vi "reportResult_getEvent.vi"(8 "error in (no error)":errorcluster, 9 "timesSuccess":i32, 10 "timesTest":i32, 11 "SalProcess in":refnum<class "SalProcess.lvclass">) -> (0 "error out":errorcluster, 3 "SalProcess out":refnum<class "SalProcess.lvclass">)   [LabVIEW 2018, in "SalProcess.lvclass"]
doc: "Report the test result of getting the event."
uses:
  SalProcess.lvclass
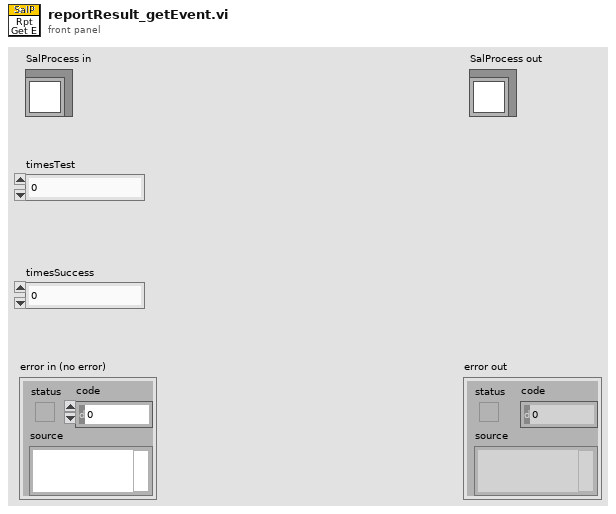
[diagram p1: front panel]
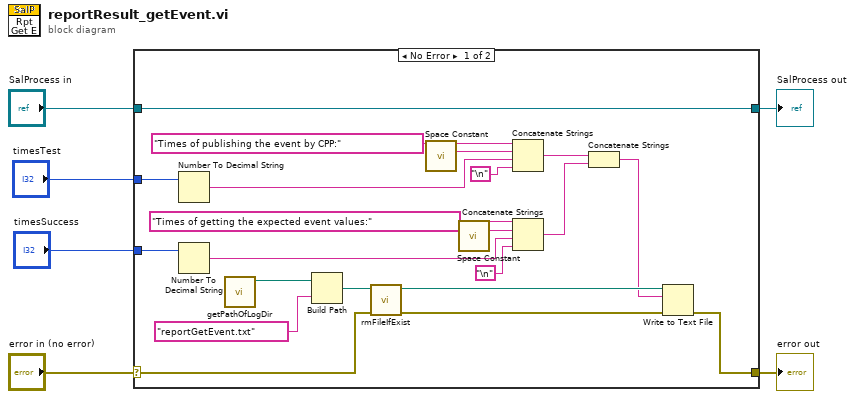
[diagram p0: block diagram]
diagram:
  n1 = case shown="No Error" "error in (no error)" {
    selector: "error in (no error)" -> [w23 w29]
    tunnel: [w7 w29] -> w5
    tunnel: [w27 w28] -> w3
    tunnel: "SalProcess in" -> [w27 w28]
    tunnel: "timesTest" -> [w22 _]
    tunnel: "timesSuccess" -> [w21 _]
    frame No Error {
      n2 = Number To Decimal String(number=w22) -> (decimal integer string=w18:string)  [unwired: 1 in]
      n3 = Number To Decimal String(number=w21) -> (decimal integer string=w14:string)  [unwired: 1 in]
      n4 = call "getPathOfLogDir.vi"() -> ("logDirPath"=w26:path)  [unwired: 11 in]
      n5 = Build Path(base path=w26, name or relative path="reportGetEvent.txt") -> (appended path=w25:path)
      n6 = call "rmFileIfExist.vi"("error in (no error)"=w23, "path"=w25) -> ("error out"=w8:errorcluster, "pathDup"=w10:path)  [unwired: 8 in]
      n7 = call <vilib>:"Space Constant.vi"() -> ("String"=w19:string)
      n8 = call <vilib>:"Space Constant.vi"() -> ("String"=w15:string)
      n9 = Concatenate Strings("Times of publishing the event by CPP:", w19, w18, "\n") -> (w12:string)
      n10 = Concatenate Strings("Times of getting the expected event values:", w15, w14, "\n") -> (w11:string)
      n11 = Concatenate Strings(w12, w11) -> (w9:string)
      n12 = Write to Text File(file (use dialog)=w10, text=w9, error in=w8) -> (error out=w7:errorcluster)  [unwired: 1 in, 2 out]
    }
    frame Error {
    }
  }
  "error out" <- w5
  "SalProcess out" <- w3
